vi "Postflight Acquisition.vi"(0 "pDataBuffer":u16[](array[numeric]), 1 "error in (no error)":errorcluster) -> (2 "pDataBuffer 2":u16[](array[numeric]), 3 "function return":i32, 4 "error out":errorcluster)   [LabVIEW 2020, in "ThorConfocal.lvlib"]
doc: "long PostflightAcquisition(char * pDataBuffer);"
uses:
  ThorConfocal.lvlib
  C:/Program Files/Thorlabs/ThorImageLS 4.1/Modules_Native/ThorConfocal.dll
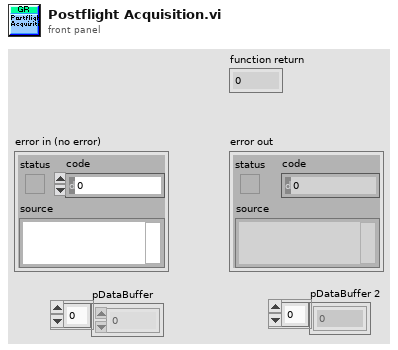
[diagram p1: front panel]
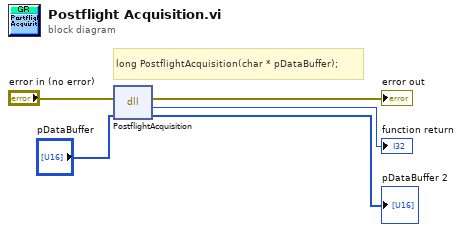
[diagram p0: block diagram]
diagram:
  # "long PostflightAcquisition(char * pDataBuffer);"
  n1 = dll-call lib="C:/Program Files/Thorlabs/ThorImageLS 4.1/Modules_Native/ThorConfocal.dll" fn="PostflightAcquisition"(error in="error in (no error)", "pDataBuffer"="pDataBuffer") -> (error out=→"error out":errorcluster, "return type"=→"function return":i32, "pDataBuffer"=→"pDataBuffer 2":u16[])  [unwired: 2 in, 1 out]
